vi "Root Locus.vi"() -> ()   [LabVIEW 2018]
uses:
  <vilib>/addons/Control Design/_Model Construction/Model Typedefs.llb/CD Transfer Function Model (SISO).ctl
  <vilib>/addons/Control Design/_Model Construction/Data Typedefs.llb/CD Root Locus with Gain Info.ctl
  <vilib>/addons/Control Design/_Model Construction/Model Typedefs.llb/CD Transfer Function Model (MIMO).ctl
  <vilib>/addons/Control Design/_Model Construction/Model Typedefs.llb/CD General Elements.ctl
  <vilib>/addons/Control Design/_Utility/Model Viewer.llb/Model Viewer SubVI/cd_Draw Transfer Function Equation (TF).vi
  <vilib>/addons/Control Design/_Dynamic Analysis/Dynamic Analysis.llb/Dynamic Analysis subVI/cd_Root Locus (Transfer Function).vi
  <vilib>/addons/Control Design/_Model Construction/NI_LinSys_Model Typedefs.lvlib
  <vilib>/addons/Control Design/_Dynamic Analysis/NI_CD_Dynamic Analysis.lvlib
  <vilib>/addons/Control Design/_Utility/NI_CD_Model Viewer.lvlib
  <vilib>/addons/Control Design/_Model Construction/NI_LinSys_Data Typedefs.lvlib
panel:
  out "Equation":picture
  in  "K1":dbl[](array[numeric]) step=0.01 format="%.2f"
  out "Root Locus Information":T1 {"Closed-Loop Poles" format="%#.2g"; "K at Bifurcation Point" format="%#.2g"; "Bifurcation Points" format="%#.2g"; "Open-Loop Poles" format="%#.2g"; "Open-Loop Zeros" format="%#.2g"}
  out "Root Locus Graph":cluster{dbl[], dbl[]}[](graph)
  in  "Transfer Function":T2[][](array[typedef]) {"delay" format="%.4f"; "Denominator" format="%#_6f"; "Numerator" format="%#.5f"}
  # "Controls Board"
  # "Root Locus Plot"
  # "b0"
  # "b1"
  # "b2"
  # "b3"
  # "a0"
  # "a1"
  # "a2"
  # "a3"
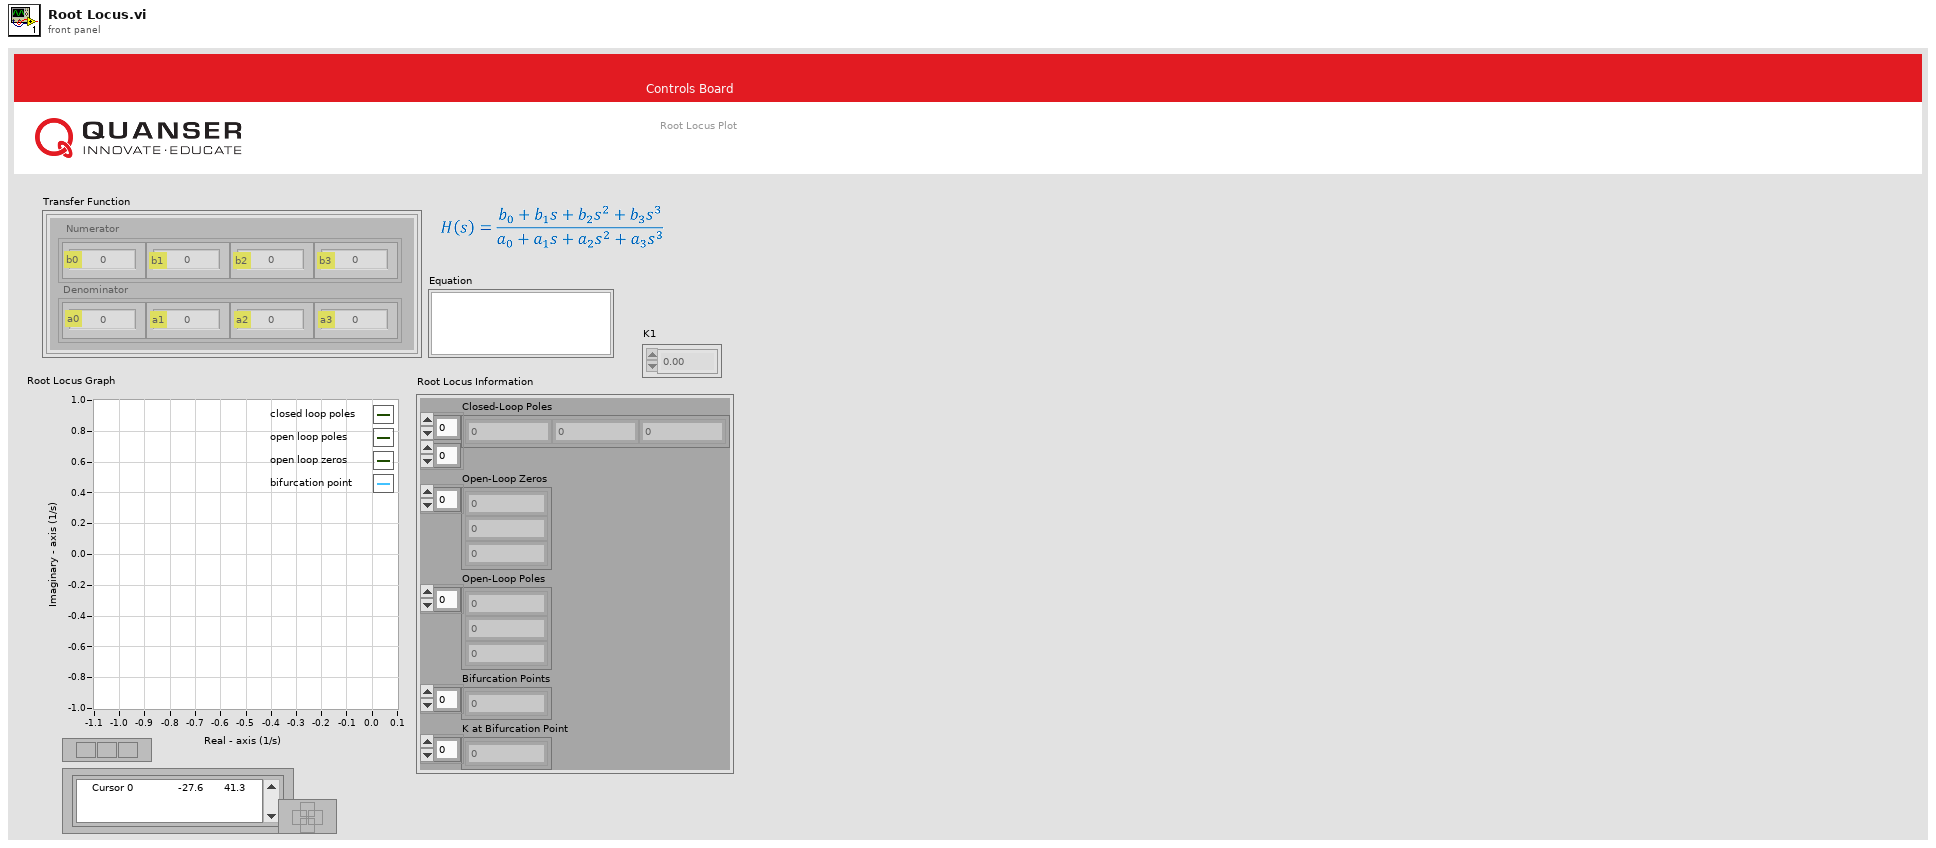
[diagram p1: front panel]
types:
  T1 = typedef "NI_LinSys_Data Typedefs.lvlib/CD Root Locus with Gain Info.ctl" = cluster{"Closed-Loop Poles":cdb[][], "Open-Loop Zeros":cdb[], "Open-Loop Poles":cdb[], "Bifurcation Points":cdb[], "K at Bifurcation Point":dbl[]}
  T2 = typedef "NI_LinSys_Model Typedefs.lvlib/CD Transfer Function Model (SISO).ctl" = cluster{"Numerator":dbl[], "Denominator":dbl[], "delay":dbl}
  T3 = typedef "NI_LinSys_Model Typedefs.lvlib/CD General Elements.ctl" = cluster{"Model name":string, "Input names":string[], "Output names":string[], "Input Delays":dbl[], "Output Delays":dbl[], "Sampling Time":dbl, "Notes":string}
  T4 = typedef "NI_LinSys_Model Typedefs.lvlib/CD Transfer Function Model (MIMO).ctl" = cluster{"properties":T3, "transfer function(s)":T2[][]}
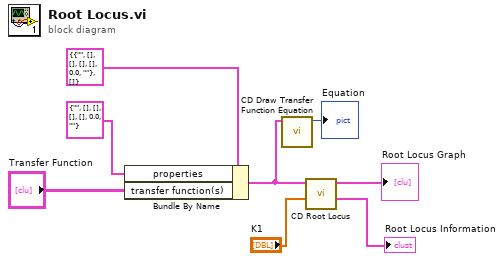
[diagram p0: block diagram]
diagram:
  n1 = Bundle By Name(cluster=T4 {"properties"={"Model name"="", "Input names"=[], "Output names"=[], "Input Delays"=[], "Output Delays"=[], "Sampling Time"=0.0, "Notes"=""}, "transfer function(s)"=[]} ("Transfer Function Model"), "properties"=T3 {"Model name"="", "Input names"=[], "Output names"=[], "Input Delays"=[], "Output Delays"=[], "Sampling Time"=0.0, "Notes"=""}, "transfer function(s)"="Transfer Function") -> (w2:T4)
  n2 = call-poly <vilib>:"CD Draw Transfer Function Equation.vi"("Transfer Function Model"=w2) -> ("Equation"=→"Equation":picture)  [unwired: 8 in, 2 out]
  n3 = call-poly <vilib>:"CD Root Locus.vi"("Gain"="K1", "Transfer Function Model"=w2) -> ("Root Locus Information"=→"Root Locus Information":T1, "Root Locus Graph"=→"Root Locus Graph":cluster{dbl[], dbl[]}[])  [unwired: 6 in, 2 out]
